vi "snap_action.vi"(0 "HGF_ImaqDx":refnum<class "HGF_ImaqDx.lvclass">, 2 "Image In":T1, 5 "error in (no error)":errorcluster, 6 "Region of Interest":i32[](array[numeric]), 7 "Step x":i32=-1, 8 "Channel":i32=-1, 9 "Step y":i32=-1) -> (14 "dup HGF_ImaqDx":refnum<class "HGF_ImaqDx.lvclass">, 16 "Image Out":T1, 19 "error out":errorcluster)   [LabVIEW 2014, in "HGF_IMAQ.lvlib" / "HGF_ImaqDx.lvclass"]
doc: "Acquires a single image into <B>Image out</B>. A snap is appropriate for low-speed or single-capture applications where ease of programming is essential."
uses:
  HGF_ImaqDx.lvclass
  <vilib>/vision/Image Controls.llb/IMAQ Image.ctl
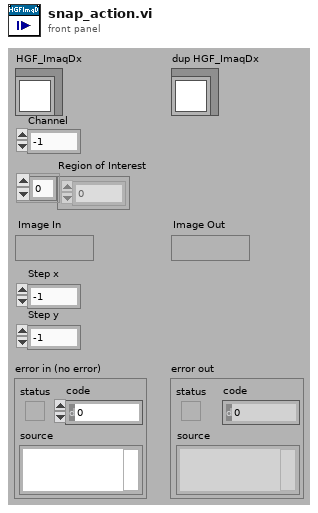
[diagram p1: front panel]
types:
  T1 = typedef "IMAQ Image.ctl" = refnum<image>
  T2 = typedef "IMAQdx.ctl" = refnum<k21>
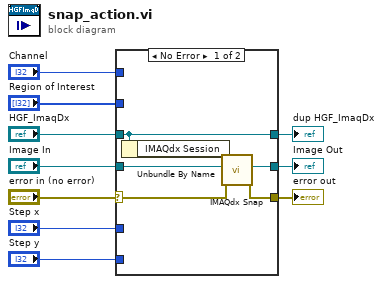
[diagram p0: block diagram]
diagram:
  n1 = case shown="No Error" "error in (no error)" {
    selector: "error in (no error)" -> [w12 w18]
    tunnel: "HGF_ImaqDx" -> [w16 w17]
    tunnel: "Image In" -> [w14 w19]
    tunnel: "Region of Interest" -> [_ _]
    tunnel: "Step x" -> [_ _]
    tunnel: "Channel" -> [_ _]
    tunnel: "Step y" -> [_ _]
    tunnel: [w15 w19] -> w4
    tunnel: [w16 w17] -> w3
    tunnel: [w11 w18] -> w1
    frame No Error {
      n2 = Unbundle By Name(w16) -> ("IMAQdx Session"=w13:T2)
      n3 = call <vilib>:"IMAQdx Snap.vi"("error in"=w12, "Image In"=w14, "Session In"=w13) -> ("error out"=w11:errorcluster, "Image Out"=w15:T1)  [unwired: 7 out]
    }
    frame Error {
    }
  }
  "error out" <- w1
  "dup HGF_ImaqDx" <- w3
  "Image Out" <- w4
